vi "niFPGA FFT Perm Buffer 512 U64.vi"(5 "x in":u64, 7 "y in":u64, 9 "stage switch":bool, 12 "Switch":bool) -> (6 "x out":u64, 8 "y out":u64)   [LabVIEW 2017]
uses:
  <vilib>/Utility/error.llb/Clear Errors.vi
  <vilib>/rvi/Emulation/niFpgaSctlEmulationGetInTimedLoop.vi
  <vilib>/rvi/DataTransferAndStorage/Container/Common/niFpgaContainerGetUniqueNameForEmu.vi
  <vilib>/rvi/DataTransferAndStorage/Container/Common/niFpgaContainerSetEmuInfo.vi
  <vilib>/rvi/eio/common/nirviEmuReportErrorAndStop.vi
  <vilib>/rvi/Memory/Memory_Emulation/nirvimemoryEmulation.vi
  <vilib>/rvi/Memory/Memory_Emulation/nirvimemoryFastEmulation.vi
  <vilib>/rvi/Memory/Memory_Emulation/niFpgaMemoryEmulationCacheClearOnFirstRun.vi
  <vilib>/rvi/Memory/Memory_Emulation/nirvimemoryEmulationManagerCache_MakeExclusive.vi
  <vilib>/rvi/Memory/Memory_Emulation/niFpgaMemoryEmulationValidateCache.vi
  <vilib>/rvi/Memory/Memory_Emulation/nirvimemoryEmulationManagerCache_InsertValue.vi
  <vilib>/rvi/Memory/Memory_Emulation/nirvimemoryEmulationManagerCache_ReleaseExclusive.vi
  <vilib>/rvi/Memory/Memory_Emulation/nirvimemoryEmulationManagerCache_GetValue.vi
  <vilib>/rvi/Emulation/niFpgaEmulationIsFPGAContextNoSignature.vi
  <vilib>/rvi/Memory/Memory_Emulation/nirvimemoryEmulationManagerCache_SetValue.vi
  <vilib>/rvi/Emulation/niFpgaSctlEmulationResourceMgr.vi
  <vilib>/rvi/LocalResourceManager/LocalResourceManager.xnode
  <vilib>/rvi/DataTransferAndStorage/Container/XNode/niFpgaContainer.xnode
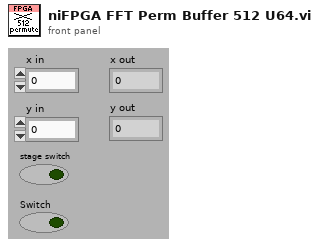
[diagram p1: front panel]
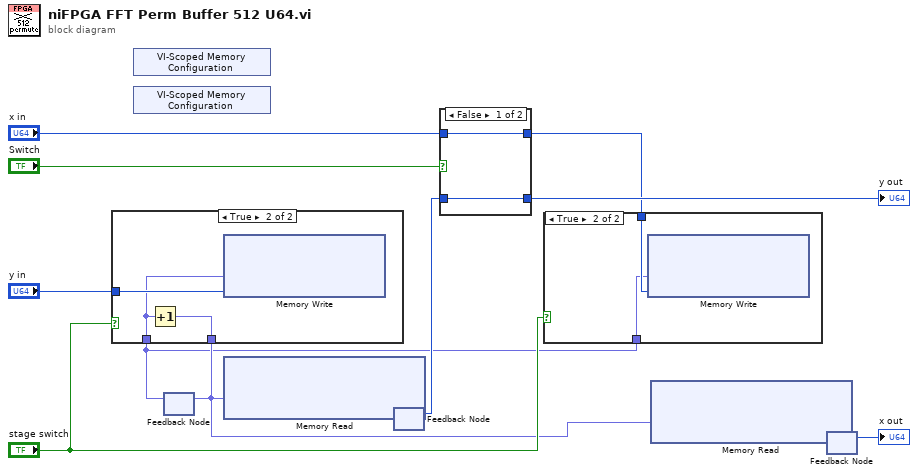
[diagram p0: block diagram]
diagram:
  n1 = xnode "VI-Scoped Memory Configuration"() -> ()  [unwired: 1 out]
  n2 = xnode "VI-Scoped Memory Configuration"() -> ()  [unwired: 1 out]
  n3 = feedback #1() -> (w1:fxp<+,9,9>)  [unwired: 1 out]
  n4 = case shown="True" "stage switch" {
    tunnel: [w13 w14] -> w2
    tunnel: w1 -> [w13 w15]
    tunnel: "y in" -> [_ w16]
    frame False {
    }
    frame True {
      n5 = Increment(x=w15) -> (x+1=w14:fxp<+,9,9>)
      n6 = xnode ("Memory Write")("Address"=w15, "Data"=w16) -> ()  [unwired: 2 out]
    }
  }
  n7 = feedback-in #1(w2) -> ()
  n8 = xnode ("Memory Read")("Address"=w2) -> ("Data"=w10:u64)  [unwired: 2 out]
  n9 = feedback-in #2(w10) -> ()
  n10 = feedback #2() -> (w4:u64)  [unwired: 1 out]
  n11 = case shown="False" "Switch" {
    tunnel: "x in" -> [w18 w20]
    tunnel: w4 -> [w17 w19]
    tunnel: [w17 w20] -> w6
    tunnel: [w18 w19] -> w5
    frame False {
    }
    frame True {
    }
  }
  "y out" <- w6
  n12 = case shown="True" "stage switch" {
    tunnel: w5 -> [_ w22]
    tunnel: w1 -> [_ w21]
    frame False {
    }
    frame True {
      n13 = xnode ("Memory Write")("Address"=w21, "Data"=w22) -> ()  [unwired: 2 out]
    }
  }
  n14 = xnode ("Memory Read")("Address"=w2) -> ("Data"=w9:u64)  [unwired: 2 out]
  n15 = feedback-in #3(w9) -> ()
  n16 = feedback #3() -> (→"x out":u64)  [unwired: 1 out]
